vi "US Data.vi"() -> ()   [LabVIEW 2016]
panel:
  in  "Average Distance":dbl
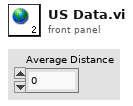
[diagram p1: front panel]
diagram:
